vi "begin.vi"() -> (0 "xgTest":u8)   [LabVIEW 2016]
uses:
  gyrosensitivities.ctl
  #defines.ctl
  GLOBALS.vi
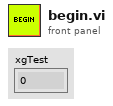
[diagram p1: front panel]
types:
  T1 = typedef "gyrosensitivities.ctl" = dbl
  T2 = typedef "#defines.ctl" = i16
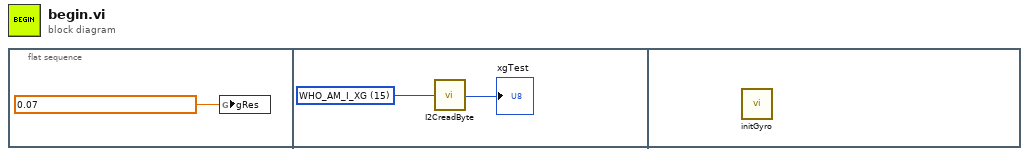
[diagram p0: block diagram]
diagram:
  n1 = flat-sequence {
    frame #0 {
      w1 = T1 0.07 items=["SENSITIVITY_GYROSCOPE_500"=0.0175, "SENSITIVITY_GYROSCOPE_2000"=0.07, "SENSITIVITY_GYROSCOPE_245"=0.00875]
      n2 = global write "GLOBALS.vi" "gRes"(w1) -> ()
    }
    frame #1 {
      w3 = T2 15 items=["CTRL_REG9_G"=35, "STATUS_REG_1"=39, "OUT_X_L_XL"=40, "FIFO_CTRL"=46, "FIFO_SRC"=47, "CTRL_REG4_G"=30, "OUT_X_L_G"=24, "OUT_TEMP_L"=21, "INT_GEN_SRC_G"=20, "ORIENT_CFG_G"=19, "CTRL_REG3_G"=18, "CTRL_REG2_G"=17, "CTRL_REG1_G"=16, "WHO_AM_I_XG"=15] ("Ring")
      n3 = call "I2CreadByte.vi"("subAddress"=w3) -> ("data"=→"xgTest":u8)
    }
    frame #2 {
      n4 = call "initGyro.vi"() -> ()  [unwired: 12 in]
    }
  }
